vi "SLSCAddToSysDef.vi"(6 "Channel":T2={"Type"=enum."Input", "Units"="", "Default Value"=0.0, "Faultable"=TRUE, "Scalable"=TRUE}, 8 "error in (no error)":errorcluster, 10 "properties":variant[](array[variant]), 11 "Section Ptr":T4 format="%.0x") -> (0 "error out":errorcluster)   [LabVIEW 2017]
uses:
  <vilib>/NI Veristand/Custom Device API/Custom Device Item Ref.ctl
  <vilib>/NI Veristand/Custom Device API/Custom Device Channel.ctl
  <vilib>/NI Veristand/Custom Device API/Custom Device Channel Type.ctl
  SLSC EDS API/JSON parsing/property.ctl
  Shared/Constants.vi
  Shared/SLSC EDS Shared.lvlib
  <vilib>/NI Veristand/Custom Device API/Custom Device API.lvlib
  <vilib>/NI Veristand/Custom Device API/Set Item Property (String).vi
panel:
  in  "property":T1
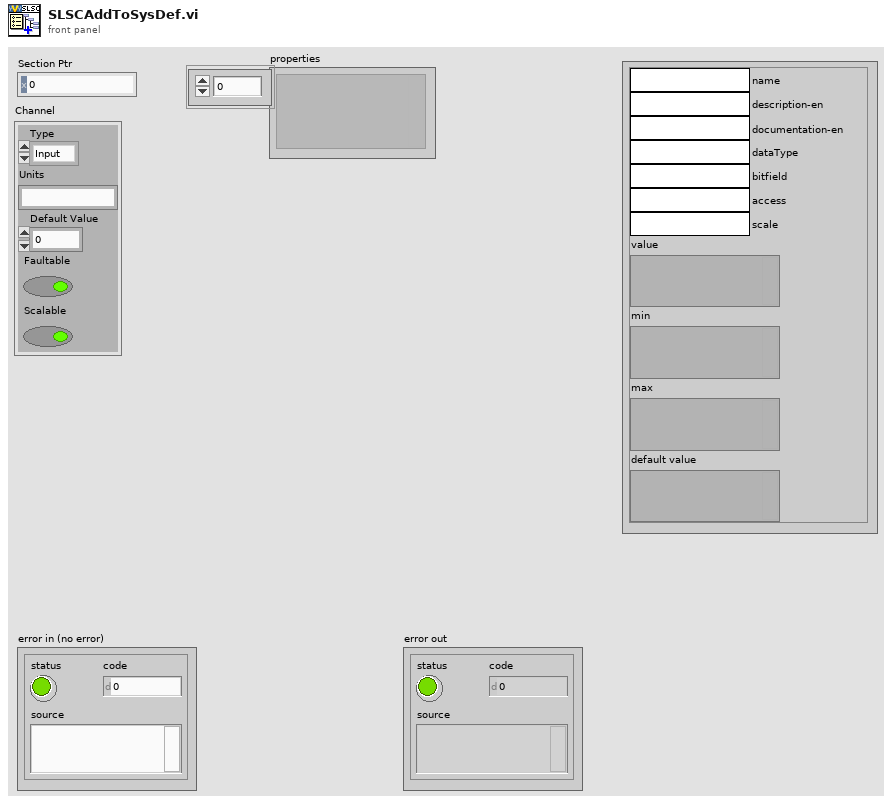
[diagram p1: front panel]
types:
  T1 = typedef "property.ctl" = cluster{"name":string, "description-en":string, "documentation-en":string, "dataType":string, "bitfield":string, "access":string, "scale":string, "value":variant, "min":variant, "max":variant, "default value":variant}
  T2 = typedef "Custom Device API.lvlib/Custom Device Channel.ctl" = cluster{"Type":T3, "Units":string, "Default Value":dbl, "Faultable":bool, "Scalable":bool}
  T3 = typedef "Custom Device API.lvlib/Custom Device Channel Type.ctl" = enum16{"Input", "Output"}
  T4 = typedef "Custom Device API.lvlib/Custom Device Item Ref.ctl" = u64
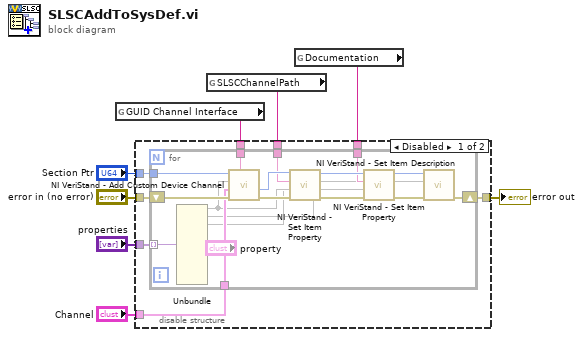
[diagram p0: block diagram]
diagram:
  n1 = global read "Constants.vi" "GUID Channel Interface"() -> (w7:string)
  n2 = global read "Constants.vi" "SLSCChannelPath"() -> (w6:string)
  n3 = global read "Constants.vi" "Documentation"() -> (w8:string)
  n4 = disable-structure shown="Disabled" {
    disable-tunnel: w8 -> [w16 _]
    disable-tunnel: w7 -> [w15 _]
    disable-tunnel: w6 -> [w14 _]
    disable-tunnel: "Channel" -> [w13 _]
    disable-tunnel: "properties" -> [w12 _]
    disable-tunnel: [w11 _] -> w3
    disable-tunnel: "Section Ptr" -> [w10 _]
    disable-tunnel: "error in (no error)" -> [w9 _]
    frame Disabled {
      n5 = for {
        tunnel: w10 -> [w29]
        shift-right: [w26] -> w11
        shift-left: w9 -> [w28]
        tunnel: w14 -> [w31]
        tunnel: w15 -> [w30]
        tunnel: w12 -> [w25] mode=indexing
        tunnel: w13 -> [w27]
        tunnel: w16 -> [w19]
        n6 = Unbundle(w25) -> (w24, w17, w18)  [unwired: 7 out]
        n7 = call <vilib>:"NI VeriStand - Add Custom Device Channel.vi"("GUID (Default Channel)"=w30, "error in (no error)"=w28, "Channel"=w27, "Channel Name"=w24, "Parent Ref in"=w29) -> ("error out"=w32:errorcluster, "Channel Ref"=w33:T4)  [unwired: 3 in, 2 out]
        n8 = call-poly <vilib>:"NI VeriStand - Set Item Property.vi"("error in (no error)"=w32, "Value"=w24, "Property Name"=w31, "Item Ref in"=w33) -> ("error out"=w22:errorcluster, "Item Ref out"=w23:T4)  [unwired: 5 in, 1 out]
        n9 = call-poly <vilib>:"NI VeriStand - Set Item Property.vi"("error in (no error)"=w22, "Value"=w18, "Property Name"=w19, "Item Ref in"=w23) -> ("error out"=w21:errorcluster, "Item Ref out"=w20:T4)  [unwired: 5 in, 1 out]
        n10 = call <vilib>:"NI VeriStand - Set Item Description.vi"("error in (no error)"=w21, "Description"=w17, "Item Ref in"=w20) -> ("error out"=w26:errorcluster)  [unwired: 6 in, 2 out]
      }
    }
    frame Enabled {
    }
  }
  "error out" <- w3
